vi "Set Units.vi"(8 "error in":errorcluster, 9 "units":T1(ring), 11 "PPT in":refnum<class "PPT.lvclass">) -> (0 "error out":errorcluster, 3 "PPT out":refnum<class "PPT.lvclass">)   [LabVIEW 2014, in "PPT Library.lvlib" / "PPT.lvclass"]
doc: "Set the units of measurement on the PPT for pressure."
uses:
  PPT.lvclass
  reusable/Session APIs/Serial/Serial Session.lvclass
  PPT.lvclass/PPT.ctl
  Configurable Device/Configurable Device.lvclass/Configurable Device.ctl
  Accessors/Read Address.vi
  Accessors/Read Serial Session.vi
  Configurable Device/Read Log Session.vi
  Configurable Device/Read ID.vi
  reusable/Session APIs/Serial/Public/Asynchronous Write.vi
  <userlib>/_Session Fwk/Session - Root.lvclass
  reusable/Session APIs/Session Log/System Log.lvclass
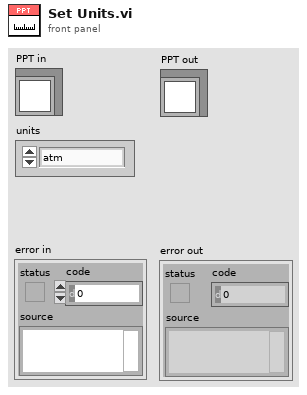
[diagram p1: front panel]
types:
  T1 = enum16{"atm", "bar", "cmwc", "ftwc", "inhg", "inwc", "kgcm", "kpa", "mbar", "mmhg", "mpa", "mwc", "psi", "user", "lcom", "pfs"}
  T2 = typedef "Session - Root.lvclass/Session Handle.ctl" = refnum<data-value>
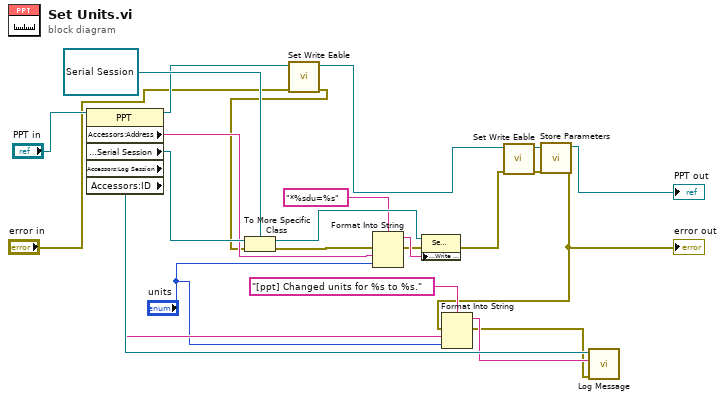
[diagram p0: block diagram]
diagram:
  n1 = property class="PPT"(reference="PPT in") -> (reference out=w4:refnum<class "PPT.lvclass">, "Accessors:Address"=w17:string, "Accessors:Serial Session"=w18:T2, "Accessors:Log Session"=w16:T2, "Accessors:ID"=w14:string)  [unwired: 1 in, 1 out]
  n2 = call "Set Write Eable.vi"("error in"="error in", "PPT in"=w4) -> ("error out"=w2:errorcluster, "PPT out"=w3:refnum<class "PPT.lvclass">)  [unwired: 8 in]
  n3 = To More Specific Class(target class=refnum<data-value> refnum, reference=w18, error in=w2) -> (specific class reference=w24:refnum<data-value>, error out=w21:errorcluster)
  n4 = Format Into String(format string="*%sdu=%s", error in=w21, w17, "units") -> (resulting string=w22:string, error out=w20:errorcluster)  [unwired: 1 in]
  n5 = property class="Serial Session"(reference=w24, error in=w20, "Public:Write - Asynchronous"=w22) -> (error out=w6:errorcluster)  [unwired: 1 out]
  n6 = call "Set Write Eable.vi"("error in"=w6, "PPT in"=w3) -> ("error out"=w10:errorcluster, "PPT out"=w9:refnum<class "PPT.lvclass">)  [unwired: 8 in]
  n7 = call "Store Parameters.vi"("error in"=w10, "PPT in"=w9) -> ("error out"=w5:errorcluster, "PPT out"=→"PPT out":refnum<class "PPT.lvclass">)  [unwired: 8 in]
  "error out" <- w5
  n8 = Format Into String(format string="[ppt] Changed units for %s to %s.", error in=w5, w14, "units") -> (resulting string=w12:string, error out=w11:errorcluster)  [unwired: 1 in]
  n9 = call "Log Message.vi"("error in"=w11, "MSG In"=w12, "session in"=w16) -> ()  [unwired: 7 in, 2 out]
